vi "Update Task Point Data.vi"(7 "Task Ident":string, 8 "error in":errorcluster, 9 "Data":variant, 10 "Point Ident":string, 11 "Series Actor in":refnum<class "Series Actor.lvclass">) -> (0 "error out":errorcluster, 3 "Series Actor out":refnum<class "Series Actor.lvclass">)   [LabVIEW 2024, in "Series Actor.lvlib" / "Series Actor.lvclass"]
uses:
  Series Actor.lvclass
  Series Actor.lvclass/Series Actor.ctl
  Task/ITask Actor/ITask Actor Messages/Update Point Data Msg/Update Point Data Msg.lvclass/Update Point Data Msg.ctl
  <vilib>/ActorFramework/Message Enqueuer/Message Enqueuer.lvclass/Message Enqueuer.ctl
  <vilib>/ActorFramework/Message Enqueuer/Enqueue.vi
  Task/ITask Actor/ITask Actor Messages/Update Point Data Msg/Update Point Data Msg.lvclass
  <vilib>/Utility/LVClass/Get LV Class Name.vi
  <resource>/AFDebug/Generate Trace for Message.vi
  <vilib>/ActorFramework/Message Priority Queue/Priority Enqueue.vi
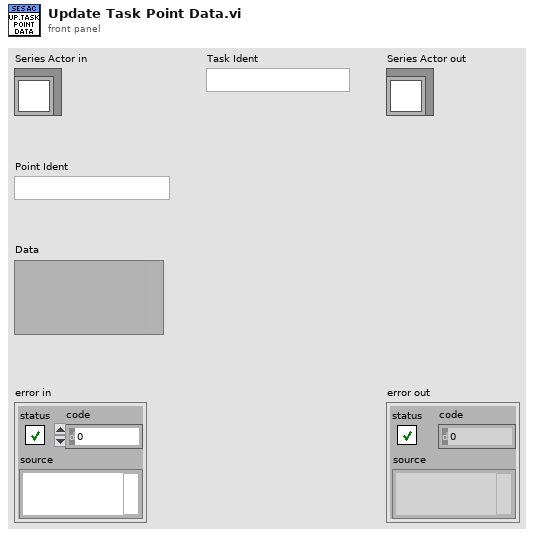
[diagram p1: front panel]
types:
  T1 = map{string, refnum<class "Message Enqueuer.lvclass">}
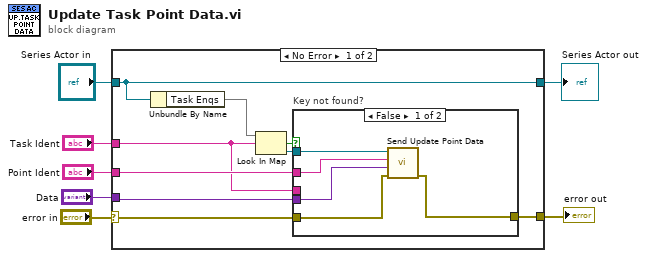
[diagram p0: block diagram]
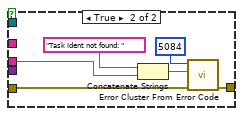
[diagram p2: hidden frame]
diagram:
  n1 = case shown="No Error" "error in" {
    selector: "error in" -> [w12 w28]
    tunnel: [w16 w29] -> w5
    tunnel: "Series Actor in" -> [w16 w29]
    tunnel: "Task Ident" -> [w8 _]
    tunnel: "Point Ident" -> [w11 _]
    tunnel: "Data" -> [w10 _]
    tunnel: [w9 w28] -> w1
    frame No Error {
      n2 = Unbundle By Name(w16) -> ("Task Enqs"=w15:T1)
      n3 = Look In Map(map=w15, key=w8) -> (key not found?=w14:bool, value=w13:refnum<class "Message Enqueuer.lvclass">)  [unwired: 1 in]
      n4 = case "Key not found?" shown="False" w14 {
        tunnel: w13 -> [w21 _]
        tunnel: w12 -> [w18 w26]
        tunnel: w11 -> [w20 _]
        tunnel: w10 -> [w19 _]
        tunnel: [w17 w27] -> w9
        tunnel: w8 -> [_ w22]
        frame False {
          n5 = call "Send Update Point Data.vi"("error in (no error)"=w18, "Data"=w19, "Point Ident"=w20, "Message Enqueuer"=w21) -> ("error out"=w17:errorcluster)  [unwired: 6 in, 1 out]
        }
        frame True {
          n6 = Concatenate Strings("Task Ident not found: " ("string"), w22) -> (w24:string)
          n7 = call <vilib>:"Error Cluster From Error Code.vi"("error in (no error)"=w26, "error message (\"\")"=w24, "error code (0)"=5084) -> ("error out"=w27:errorcluster)  [unwired: 6 in]
        }
      }
    }
    frame Error {
    }
  }
  "error out" <- w1
  "Series Actor out" <- w5
